vi "SeCrTs-DI Index Element.vi"(8 "Storage Index":i32[](array[numeric]), 9 "Write/Read":enum16{"Write", "Read"}(ring)=enum."Read", 11 "Pumb Index":i32[](array[numeric])) -> (0 "Storage Index":i32[](array[numeric]), 3 "Pumb index":i32[](array[numeric]))   [LabVIEW 2022 SP3]
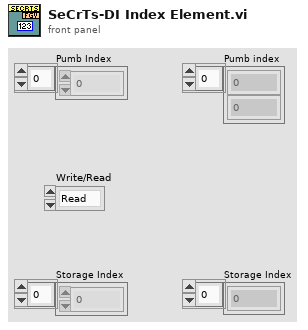
[diagram p1: front panel]
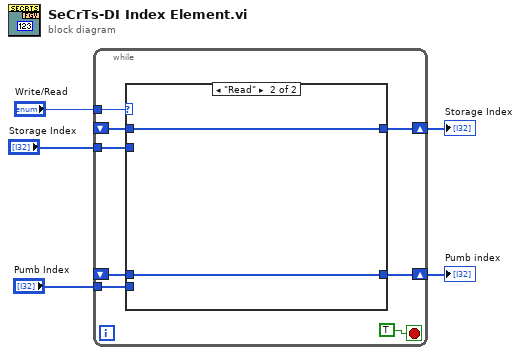
[diagram p0: block diagram]
diagram:
  n1 = while {
    tunnel: "Write/Read" -> [w12]
    shift-right: [w11] -> w3
    shift-left: _ -> [w10]
    tunnel: "Pumb Index" -> [w9]
    tunnel: "Storage Index" -> [w8]
    shift-right: [w7] -> w1
    shift-left: _ -> [w6]
    stop <- TRUE stop-if-true
    n2 = case shown="\"Read\"" w12 {
      tunnel: [w15 w17] -> w11
      tunnel: w10 -> [_ w17]
      tunnel: w9 -> [w15 _]
      tunnel: w8 -> [w14 _]
      tunnel: [w14 w16] -> w7
      tunnel: w6 -> [_ w16]
      frame "Write" {
      }
      frame "Read" {
      }
    }
  }
  "Pumb index" <- w3
  "Storage Index" <- w1
